vi "Integral.vi"(8 "error in (no error)":errorcluster, 11 "Tested Signals":dynamicdata(waveform)) -> (0 "error out":errorcluster, 3 "Integral":dbl)   [LabVIEW 2011]
doc: "Example of the SubVI with Error Handling template.\n\nThis VI is used as a subvi in the Limit Example.vi (Example of the use of Single Loop Application template). If there is no error this VI calculates the area of the signal that is under/over the +-5 band. \n\nIf there is an error, then it outputs 0."
uses:
  Instance           2 16Saved   Integral .vi
  Instance           1 16Saved   Integral .vi
panel:
  # "Go to File»VI Properties»Documentation for a detailed explanation of this VI"
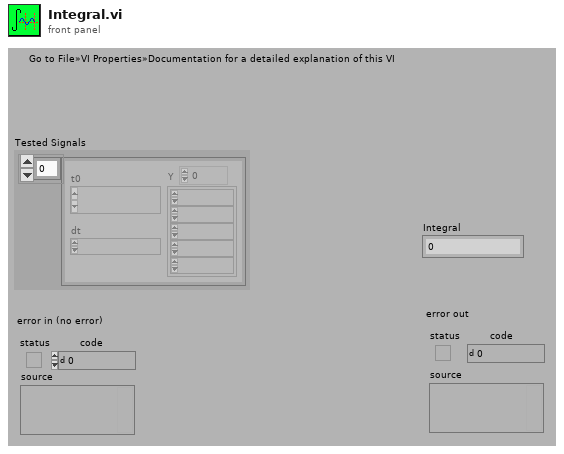
[diagram p1: front panel]
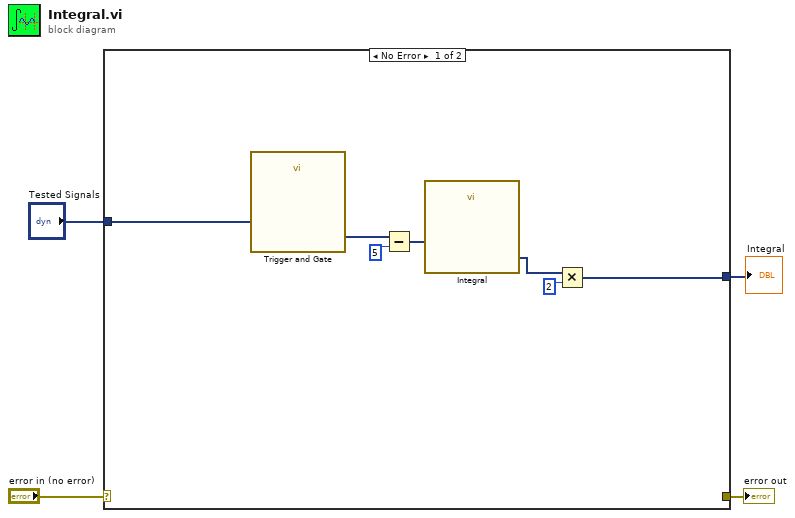
[diagram p0: block diagram]
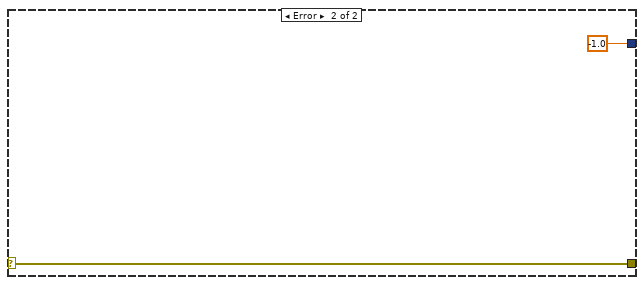
[diagram p2: hidden frame]
diagram:
  n1 = case shown="No Error" "error in (no error)" {
    selector: "error in (no error)" -> [_ w12]
    tunnel: [_ w12] -> w3
    tunnel: [w7 -1.0] -> w2
    tunnel: "Tested Signals" -> [w6 _]
    frame No Error {
      n2 = call "Trigger and Gate"("Signals"=w6) -> ("Triggered Signals"=w8:dynamicdata)  [unwired: 7 in, 3 out]
      n3 = Subtract(x=w8, y=5) -> (x-y=w10:dynamicdata)
      n4 = call "Integral"("Signals"=w10) -> ("Result"=w5:dynamicdata)  [unwired: 5 in, 1 out]
      n5 = Multiply(x=w5, y=2) -> (x*y=w7:dynamicdata)
    }
    frame Error {
    }
  }
  "error out" <- w3
  "Integral" <- w2
